vi "Initialize.vi"(7 "IP":string="//localhost", 8 "error in (no error)":errorcluster, 9 "Image Name":string="CH1", 10 "Night Directory:":string="C:\\Users\\observer\\Desktop\\Imagens", 11 "SPARC4_GUI in":refnum<class "SPARC4_GUI.lvclass">) -> (0 "error out":errorcluster, 3 "SPARC4_GUI out":refnum<class "SPARC4_GUI.lvclass">)   [LabVIEW 2018, in "SPARC4_GUI.lvclass"]
uses:
  SPARC4_GUI.lvclass
  Channel GUI/Channel GUI.lvclass
  Channel GUI/Channel GUI.lvclass/Channel GUI.ctl
  SPARC4_GUI.lvclass/SPARC4_GUI.ctl
  State Machine/State Machine.lvclass
panel:
  in  "Channel GUI.lvclass":refnum<class "Channel GUI.lvclass">
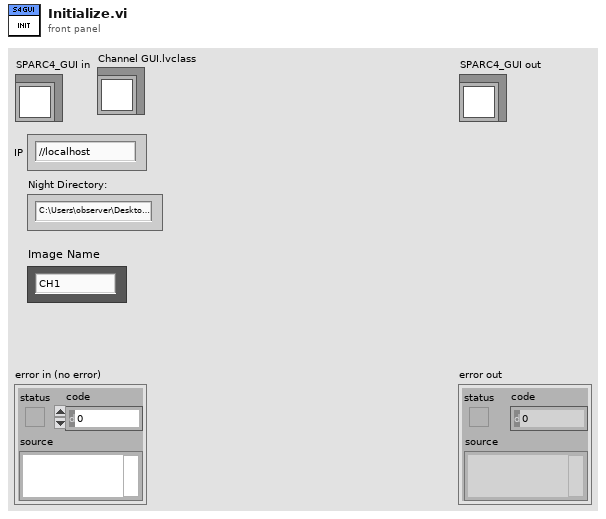
[diagram p1: front panel]
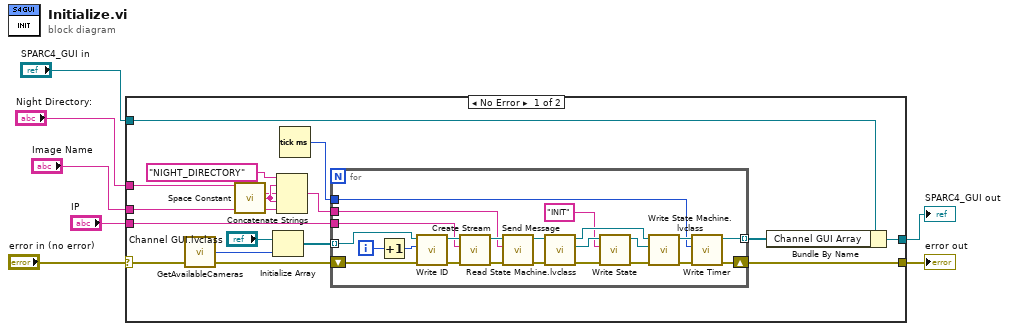
[diagram p0: block diagram]
diagram:
  n1 = case shown="No Error" "error in (no error)" {
    selector: "error in (no error)" -> [w16 w48]
    tunnel: [w9 w48] -> w6
    tunnel: [w12 w47] -> w4
    tunnel: "SPARC4_GUI in" -> [w13 w47]
    tunnel: "Image Name" -> [w21 _]
    tunnel: "Night Directory:" -> [w20 _]
    tunnel: "IP" -> [w15 _]
    frame No Error {
      n2 = call <userlib>:"GetAvailableCameras.vi"("error in (no error)"=w16) -> ("error out"=w17:errorcluster, "totalCameras"=w8:i32)  [unwired: 2 in, 1 out]
      n3 = call <vilib>:"Space Constant.vi"() -> ("String"=w22:string)
      n4 = Initialize Array("Channel GUI.lvclass", w8) -> (w18:refnum<class "Channel GUI.lvclass">[])
      n5 = Concatenate Strings("NIGHT_DIRECTORY" ("Message"), w22, w20, w22, w21) -> (w14:string)
      n6 = Tick Count (ms)() -> (millisecond timer value=w11:u32)
      n7 = for {
        shift-right: [w24] -> w9
        shift-left: w17 -> [w44]
        tunnel: w18 -> [w45] mode=indexing
        tunnel: w15 -> [w38]
        tunnel: w14 -> [w37]
        tunnel: w11 -> [w26]
        tunnel: [w25] -> w10 mode=indexing
        i -> [w46]
        n8 = Increment(x=w46) -> (x+1=w43:i32)
        n9 = call "Write ID.vi"("error in (no error)"=w44, "ID"=w43, "Channel GUI in"=w45) -> ("error out"=w42:errorcluster, "Channel GUI out"=w41:refnum<class "Channel GUI.lvclass">)  [unwired: 7 in]
        n10 = call "Create Stream.vi"("error in (no error)"=w42, "IP"=w38, "Channel GUI in"=w41) -> ("error out"=w39:errorcluster, "Channel GUI out"=w40:refnum<class "Channel GUI.lvclass">)  [unwired: 7 in]
        n11 = call "Send Message.vi"("error in (no error)"=w39, "Message"=w37, "Channel GUI in"=w40) -> ("error out"=w35:errorcluster, "Channel GUI out"=w36:refnum<class "Channel GUI.lvclass">)  [unwired: 7 in]
        n12 = call "Read State Machine.lvclass.vi"("error in (no error)"=w35, "Channel GUI in"=w36) -> ("error out"=w31:errorcluster, "State Machine.lvclass"=w34:refnum<class "State Machine.lvclass">, "Channel GUI out"=w32:refnum<class "Channel GUI.lvclass">)  [unwired: 7 in]
        n13 = call-dynamic "Write State.vi"("error in (no error)"=w31, "State"="INIT", "State Machine in"=w34) -> ("error out"=w30:errorcluster, "State Machine out"=w33:refnum<class "State Machine.lvclass">)  [unwired: 7 in]
        n14 = call "Write State Machine.lvclass.vi"("error in (no error)"=w30, "State Machine.lvclass"=w33, "Channel GUI in"=w32) -> ("error out"=w27:errorcluster, "Channel GUI out"=w28:refnum<class "Channel GUI.lvclass">)  [unwired: 7 in]
        n15 = call "Write Timer.vi"("error in (no error)"=w27, "Timer"=w26, "Channel GUI in"=w28) -> ("error out"=w24:errorcluster, "Channel GUI out"=w25:refnum<class "Channel GUI.lvclass">)  [unwired: 7 in]
      }
      n16 = Bundle By Name(cluster=w13, "Channel GUI Array"=w10) -> (w12:refnum<class "SPARC4_GUI.lvclass">)
    }
    frame Error {
    }
  }
  "error out" <- w6
  "SPARC4_GUI out" <- w4
